vi "DRC91SetHeatRange.vi"(0 "VISA Rsrc":refnum<visa-resource-name>="GPIB0::12::INSTR", 5 "HtrRange":u16(ring) caption="Échelle de chauffage" items=["Off"=1, "-3 Low"=2, "-2 Med"=3, "-1 High"=4, "Max"=5], 11 "error in":errorcluster) -> (15 "error out":errorcluster)   [LabVIEW 2010]
doc: "Ce Vi interroge l'instrument sur l'échelle de chauffage en watt et le pourcentage de chauffage actuel et retourne une puissance de chauffage en Watts"
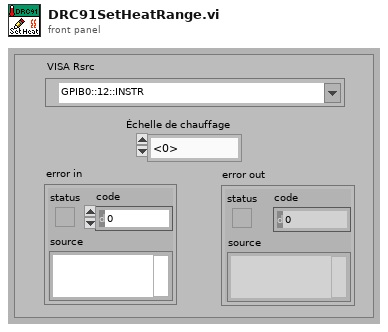
[diagram p1: front panel]
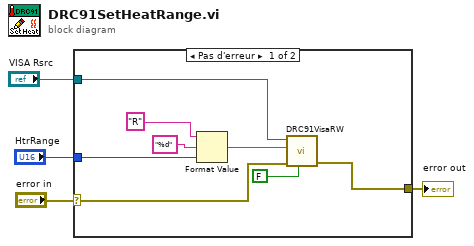
[diagram p0: block diagram]
diagram:
  n1 = case shown="Pas d'erreur" "error in" {
    selector: "error in" -> [w11 w13]
    tunnel: [w5 w13] -> w4
    tunnel: "VISA Rsrc" -> [w12 _]
    tunnel: "HtrRange" -> [w9 _]
    frame No Error {
      n2 = Format Value(string ("")="R", format string="%d", value (0)=w9) -> (output string=w6:string)
      n3 = call <userlib>:"DRC91VisaRW.vi"("Lecture?(T)"=FALSE, "error in (no error)"=w11, "ChaineCom"=w6, "VISA Rsrc"=w12) -> ("error out"=w5:errorcluster)  [unwired: 3 in, 3 out]
    }
    frame Error {
    }
  }
  "error out" <- w4
